vi "Write_binary_file.vi"(8 "string 2":string, 9 "output bit stream 3":i8[](array[numeric]) caption="output bit stream", 10 "Save path":path) -> ()   [LabVIEW 2014]
panel:
  out "string":string
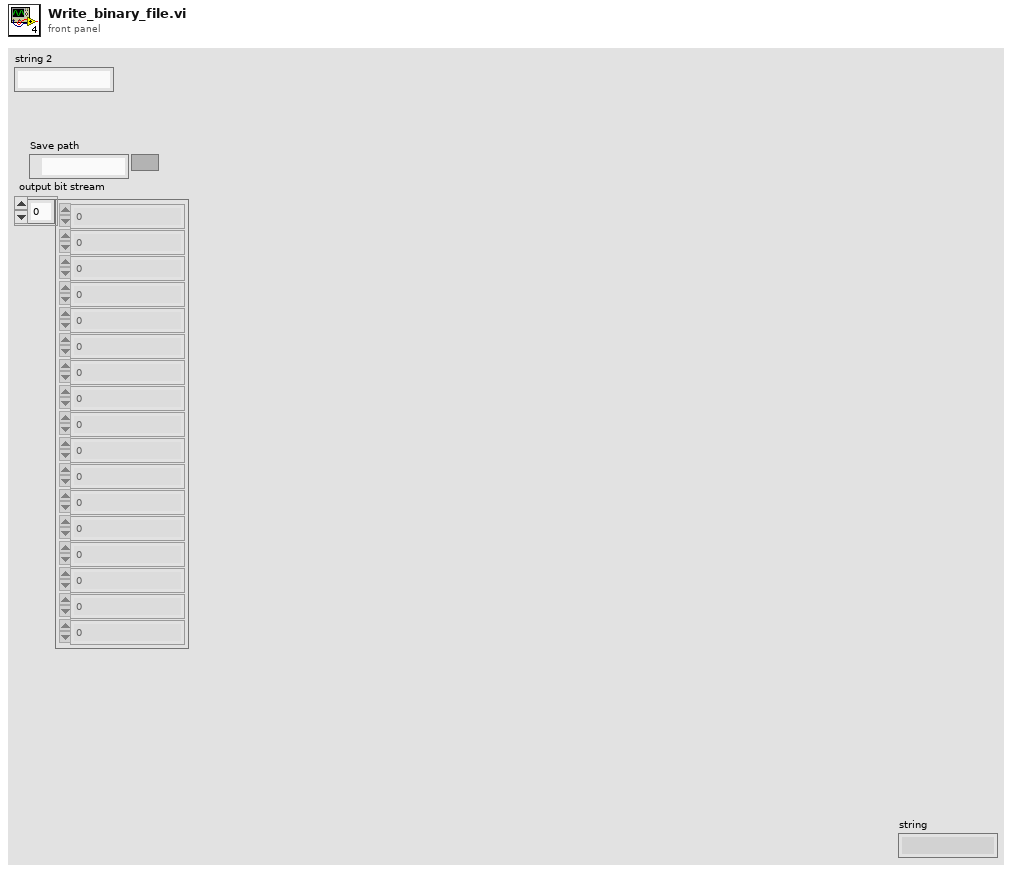
[diagram p1: front panel]
types:
  T1 = enum16{"big-endian, network order", "native, host order", "little-endian"}
  T2 = enum16{"open", "replace", "create", "open or create", "replace or create", "replace or create with confirmation"}
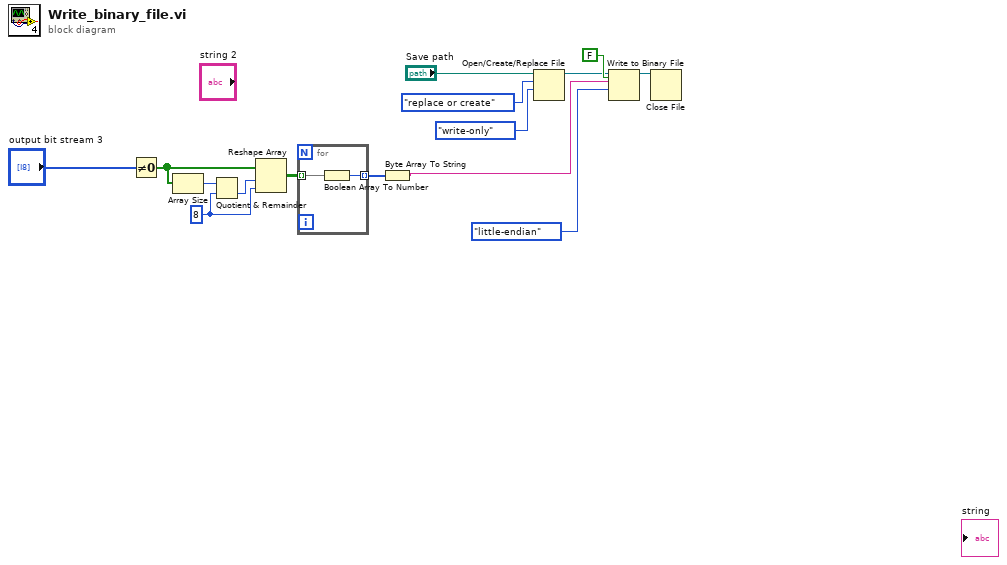
[diagram p0: block diagram]
diagram:
  w4 = 8
  n1 = Not Equal To 0?(x="output bit stream 3") -> (x != 0?=w7:bool[])
  n2 = Array Size(array=w7) -> (size(s)=w5:i32)
  n3 = Quotient & Remainder(x=w5, y=w4) -> (floor(x/y)=w3:i32)  [unwired: 1 out]
  n4 = Reshape Array(w7, w3, w4) -> (w6:bool[][])
  n5 = for {
    tunnel: [w17] -> w8 mode=indexing
    tunnel: w6 -> [w16] mode=indexing
    n6 = Boolean Array To Number(Boolean array=w16) -> (number=w17:u32)
  }
  n7 = Byte Array To String(unsigned byte array=w8) -> (string=w1:string)
  n8 = Open/Create/Replace File(file path (use dialog)="Save path", operation (0:open)=T2."replace or create", access (0:read/write)=enum16{"read/write", "read-only", "write-only"}."write-only") -> (refnum out=w10:refnum<file>)  [unwired: 3 in, 2 out]
  n9 = Write to Binary File(file (use dialog)=w10, data=w1, 5:FALSE ("prepend array or string size? (T)"), 9:T1."little-endian" ("byte order (0:big-endian, network order)")) -> (refnum out=w9:refnum<file>)  [unwired: 2 in, 2 out]
  n10 = Close File(refnum=w9) -> ()  [unwired: 1 in, 2 out]
